vi "Flag_for_ReLinking.vi"(8 "error in (no error)":errorcluster, 10 "relink":bool, 11 "AB_Source_VI in":refnum<class "AB_Source_VI.lvclass">) -> (0 "error out":errorcluster, 3 "AB_Source_VI out":refnum<class "AB_Source_VI.lvclass">)   [LabVIEW 2020, in "AB_Source_VI.lvclass"]
uses:
  <vilib>/AppBuilder/AB_Classes/Source/VI/AB_Source_VI.lvclass
  <vilib>/AppBuilder/AB_Classes/Source/VI/AB_Source_VI.lvclass/AB_Source_VI.ctl
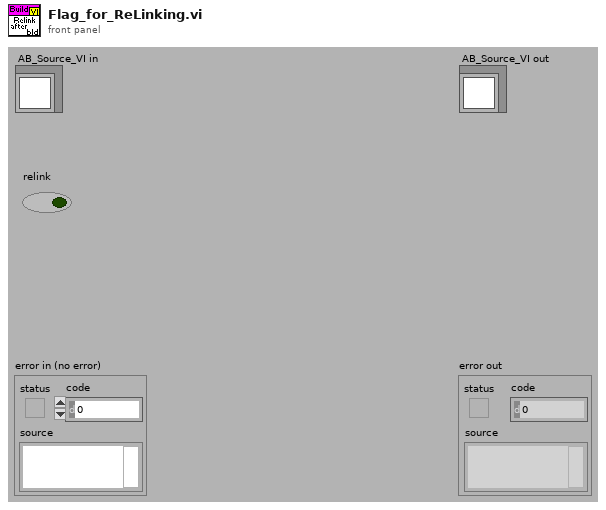
[diagram p1: front panel]
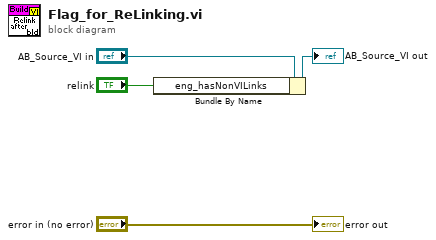
[diagram p0: block diagram]
diagram:
  n1 = Bundle By Name(cluster="AB_Source_VI in", "eng_hasNonVILinks"="relink") -> (→"AB_Source_VI out":refnum<class "AB_Source_VI.lvclass">)
  "error out" <- "error in (no error)"
